vi "SLSC Convert SLSC Channel Path into Tree Tag.vi"(11 "SLSC Channel Path":string) -> (2 "Status?":bool, 3 "Tree Item Channel":string)   [LabVIEW 2019, in "SLSC CD Shared.lvlib"]
uses:
  SLSC CD Shared.lvlib
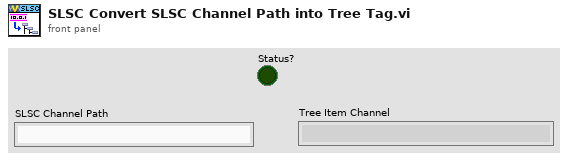
[diagram p1: front panel]
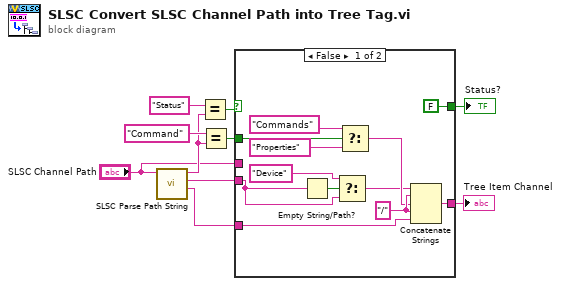
[diagram p0: block diagram]
diagram:
  n1 = call "SLSC Parse Path String.vi"("SLSC Channel Path"="SLSC Channel Path") -> ("Property or Command"=w10:string, "Physical Channel"=w9:string, "Datatype"=w5:string)  [unwired: 7 in, 1 out]
  n2 = Equal?(x="Status", y=w5) -> (x = y?=w3:bool)
  n3 = Equal?(x="Command", y=w5) -> (x = y?=w7:bool)
  n4 = case shown="False" w3 {
    selector: w3 -> [_ w23]
    tunnel: w10 -> [w22 _]
    tunnel: w9 -> [w21 _]
    tunnel: [w19 w24] -> w8
    tunnel: w7 -> [w15 _]
    tunnel: "SLSC Channel Path" -> [_ w24]
    tunnel: [FALSE w23] -> w1
    frame False {
      w18 = "/" ("string")
      n5 = Empty String/Path?(string/path=w21) -> (empty?=w12:bool)
      n6 = Select(t="Device" ("before match"), s=w12, f=w21) -> (s? t:f=w13:string)
      n7 = Select(t="Commands" ("x"), s=w15, f="Properties") -> (s? t:f=w17:string)
      n8 = Concatenate Strings(w13, w18, w17, w18, w22) -> (w19:string)
    }
    frame True {
      # "Special channels for EDS CD"
    }
  }
  "Tree Item Channel" <- w8
  "Status?" <- w1
